vi "Log Error to DS.vi"(11 "Text Logged to DS Log":string) -> (0 "Error Out":errorcluster)   [LabVIEW 2017]
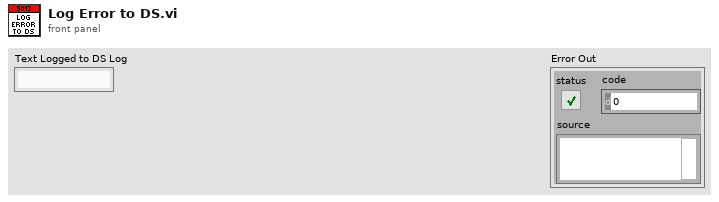
[diagram p1: front panel]
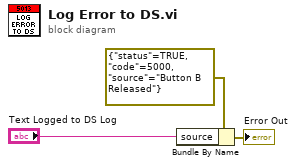
[diagram p0: block diagram]
diagram:
  n1 = Bundle By Name(cluster=errorcluster {"status"=TRUE, "code"=5000, "source"="Button B Released"} ("error constant"), "source"="Text Logged to DS Log") -> (→"Error Out":errorcluster)
